vi "Acceleration mMc Edited.vi"(0 "accel in":dbl, 1 "Port":T1={"P type"=0, "reference"="", " Terminator "="\r\n", "Timeout"=300} {"Timeout" step=10; "P type" items=["none", "RS-232C"]}, 3 "error in (no error)":errorcluster, 4 "set/get":bool caption="set\n\n\nget", 5 "Controller #":string) -> (6 "accel out":dbl, 9 "error out":errorcluster)   [LabVIEW 2021]
panel:
  # "Acceleration"
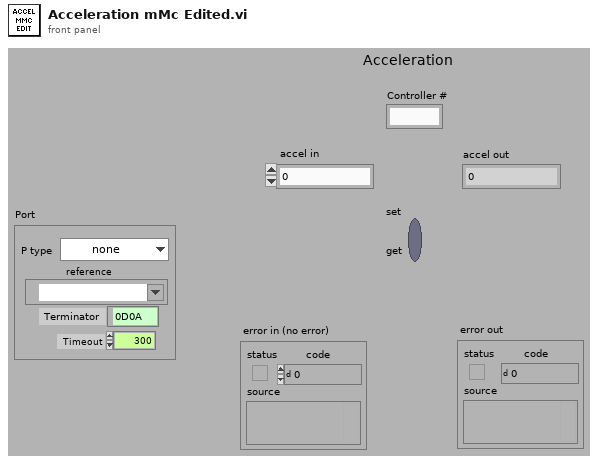
[diagram p1: front panel]
types:
  T1 = cluster{"P type":u16, "reference":refnum<visa-resource-name>, " Terminator ":string, "Timeout":i32}
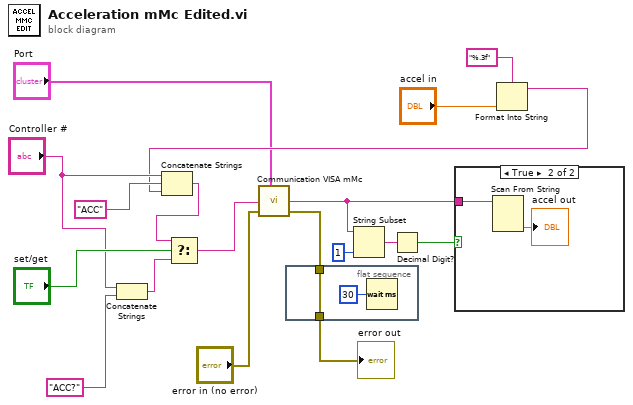
[diagram p0: block diagram]
diagram:
  n1 = Concatenate Strings("Controller #", "ACC?") -> (w18:string)
  n2 = flat-sequence {
    tunnel: [w20] -> w2
    tunnel: w1 -> [w20]
    frame #0 {
      n3 = Wait (ms)(milliseconds to wait=u32 30) -> ()  [unwired: 1 out]
    }
  }
  n4 = Format Into String(format string="%.3f", "accel in") -> (resulting string=w8:string)  [unwired: 2 in, 1 out]
  n5 = Concatenate Strings("Controller #", "ACC", w8) -> (w16:string)
  n6 = Select(t=w16, s="set/get", f=w18) -> (s? t:f=w15:string)
  n7 = call "Communication VISA mMc.vi"("Port"="Port", "Command"=w15, "error in (no error)"="error in (no error)") -> ("Return"=w7:string, "error out"=w1:errorcluster)  [unwired: 3 in, 2 out]
  n8 = String Subset(string=w7, length (rest)=1 ("length (rest)")) -> (substring=w5:string)  [unwired: 1 in]
  n9 = Decimal Digit?(1:w5) -> (0:w4:bool)
  n10 = case shown="True" w4 {
    tunnel: w7 -> [_ w21]
    frame False {
    }
    frame True {
      n11 = Scan From String(input string=w21) -> (output 1=→"accel out":dbl)  [unwired: 4 in, 3 out]
    }
  }
  "error out" <- w2
